vi "Set Angle.vi"(4 "Axis":T1, 8 "error in (no error)":errorcluster, 10 "Angle (°)":dbl, 11 "instrument.PPMS2 in":refnum<class "instrument.PPMS2.lvclass">) -> (0 "error out":errorcluster, 3 "instrument.PPMS2 out":refnum<class "instrument.PPMS2.lvclass">)   [LabVIEW 2016, in "instrument.PPMS2.lvclass"]
uses:
  instrument.PPMS2.lvclass
  <userlib>/LevyLab/Levylab Instruments/Instrument Types/Cryostat/Typedefs/Rotator Axis--Enum.ctl
  <userlib>/LevyLab/Levylab Instruments/Instrument Types/Cryostat/Instrument.Cryostat.lvclass
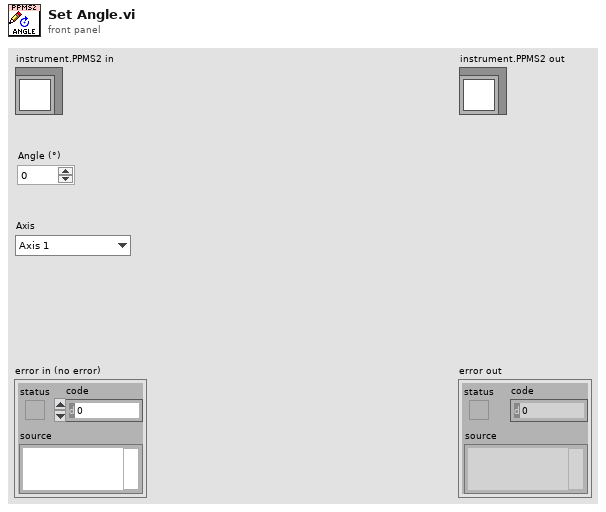
[diagram p1: front panel]
types:
  T1 = typedef "Instrument.Cryostat.lvclass/Rotator Axis--Enum.ctl" = enum16{"Axis 1", "Axis 2"}
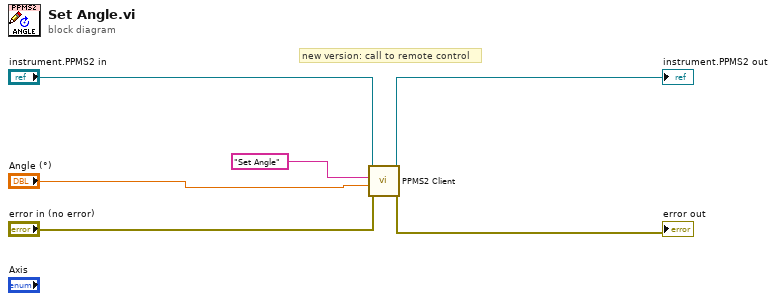
[diagram p0: block diagram]
diagram:
  # "new version: call to remote control"
  n1 = call "PPMS2 Client.vi"("error in (no error)"="error in (no error)", "Data"="Angle (°)", "Command"="Set Angle", "instrument.PPMS2 in"="instrument.PPMS2 in") -> ("error out"=→"error out":errorcluster, "instrument.PPMS2 out"=→"instrument.PPMS2 out":refnum<class "instrument.PPMS2.lvclass">)  [unwired: 4 in, 2 out]
